vi "CartesianToPolar.vi"(10 "y":dbl, 11 "x":dbl) -> (2 "theta (radians)":dbl, 3 "r":dbl)   [LabVIEW 2013]
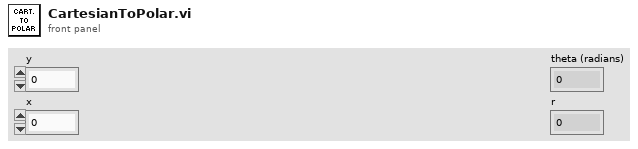
[diagram p1: front panel]
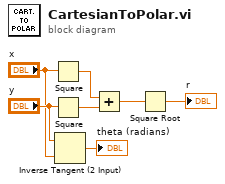
[diagram p0: block diagram]
diagram:
  n1 = Square(x="x") -> (x^2=w5:dbl)
  n2 = Square(x="y") -> (x^2=w4:dbl)
  n3 = Inverse Tangent (2 Input)(1:"x", 2:"y") -> (0:→"theta (radians)":dbl)
  n4 = Add(x=w5, y=w4) -> (x+y=w6:dbl)
  n5 = Square Root(x=w6) -> (sqrt(x)=→"r":dbl)
